vi "Fdx Create Udp Port (RX-SAP).vi"(8 "error in (no error)":errorcluster, 9 "VlId":u16, 10 "SapPort Config":T2, 11 "port handle in":u32) -> (0 "error out":errorcluster, 1 "computedAddresses":T1 {"MACsrc" format="%.0x"}, 2 "sapPort handle out":u32, 3 "port handle out":u32)   [LabVIEW 2020, in "AIM664LV.lvlib"]
doc: "Creates a port to receive data from a specified SAP connectionless port. This function can be used only, if receiver is not running. This function assumes that FdxCmdRxVLControl was previously called in order to enable a VL for reception. On this VL this function creates an AFDX SAP Rx-port."
uses:
  AIM664LV.lvlib
  _controls/sap_config_rx.ctl
  _controls/comm_computedMAC-IP.ctl
  helpers/EthFrameManagement/EthFrameManagement.lvlib
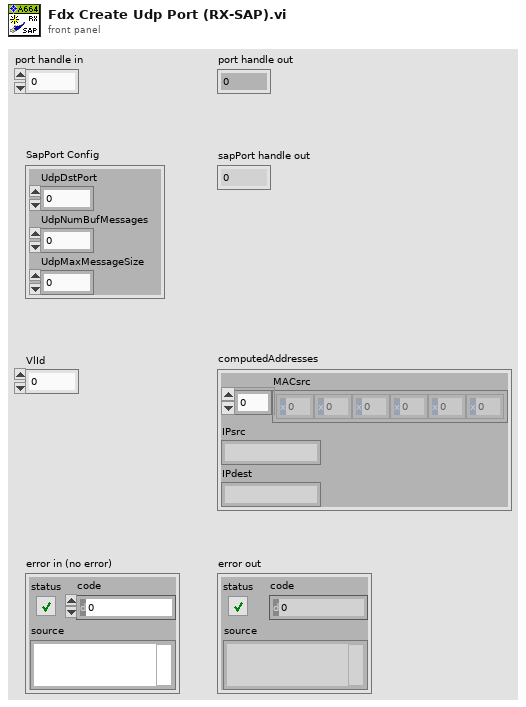
[diagram p1: front panel]
types:
  T1 = typedef "AIM664LV.lvlib/comm_computedMAC-IP.ctl" = cluster{"MACsrc":u8[], "IPsrc":string, "IPdest":string}
  T2 = typedef "AIM664LV.lvlib/sap_config_rx.ctl" = cluster{"UdpDstPort":u16, "UdpNumBufMessages":u32, "UdpMaxMessageSize":u32}
  T3 = cluster{"UdpDst":u32, "IpDst":u32, "VlId":u32, "UdpNumBufMessages":u32, "UdpMaxMessageSize":u32}
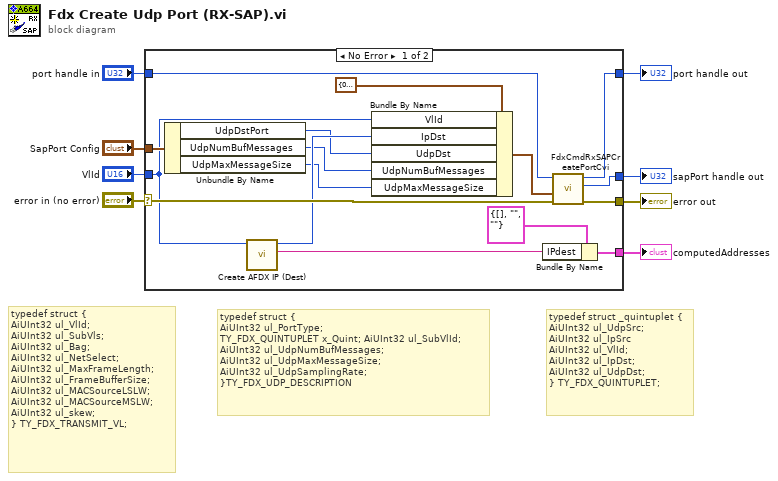
[diagram p0: block diagram]
diagram:
  # "typedef struct _quintuplet {\nAiUInt32 ul_UdpSrc;\nAiUInt32 ul_IpSrc\nAiUInt32 ul_VlId;\nAiUInt32 ul_IpDst;\nAiUInt32 ul_UdpDst;\n} TY_FDX_QUINTUPLET;"
  # "typedef struct {\nAiUInt32 ul_PortType;\nTY_FDX_QUINTUPLET x_Quint; AiUInt32 ul_SubVlId;\nAiUInt32 ul_UdpNumBufMessages;\nAiUInt32 ul_UdpMaxMessageSize;\nAiUInt32 ul_UdpSamplingRate;\n}TY_FDX_UDP_DESCRIPTION"
  # "typedef struct {\nAiUInt32 ul_VlId;\nAiUInt32 ul_SubVls;\nAiUInt32 ul_Bag;\nAiUInt32 ul_NetSelect;\nAiUInt32 ul_MaxFrameLength;\nAiUInt32 ul_FrameBufferSize;\nAiUInt32 ul_MACSourceLSLW;\nAiUInt32 ul_MACSourceMSLW;\nAiUInt32 ul_skew;\n} TY_FDX_TRANSMIT_VL;"
  n1 = case shown="No Error" "error in (no error)" {
    selector: "error in (no error)" -> [w23 w25]
    tunnel: "port handle in" -> [w24 w26]
    tunnel: [w10 w26] -> w6
    tunnel: [w19 w25] -> w5
    tunnel: "SapPort Config" -> [w22 _]
    tunnel: [w21 _] -> w3
    tunnel: "VlId" -> [w20 _]
    tunnel: [w9 _] -> w1
    frame No Error {
      n2 = Unbundle By Name(w22) -> ("UdpDstPort"=w14:u16, "UdpNumBufMessages"=w13:u32, "UdpMaxMessageSize"=w12:u32)
      n3 = call "Create AFDX IP (Dest).vi"("VL"=w20) -> ("ip string"=w11:string, "ip net"=w15:u32)  [unwired: 9 in]
      n4 = Bundle By Name(cluster=T3 {"UdpDst"=0, "IpDst"=0, "VlId"=0, "UdpNumBufMessages"=0, "UdpMaxMessageSize"=0} ("SapCreateIn"), "VlId"=w20, "IpDst"=w15, "UdpDst"=w14, "UdpNumBufMessages"=w13, "UdpMaxMessageSize"=w12) -> (w17:T3)
      n5 = Bundle By Name(cluster=T1 {"MACsrc"=[], "IPsrc"="", "IPdest"=""} ("computedAddresses"), "IPdest"=w11) -> (w21:T1)
      n6 = call "FdxCmdRxSAPCreatePortCvi.vi"("error in"=w23, "SapCreateIn"=w17, "InstrumentHandle_port"=w24) -> ("error out"=w19:errorcluster, "UdpHandle"=w9:u32, "InstrumentHandle_port"=w10:u32)  [unwired: 6 in]
    }
    frame Error {
    }
  }
  "port handle out" <- w6
  "sapPort handle out" <- w1
  "error out" <- w5
  "computedAddresses" <- w3
